vi "ReadDefaultConfigurationFile.vi"(8 "error in (no error)":errorcluster, 11 "SMO.UI.MAUI in":refnum<class "SMO.UI.MAUI.lvclass">) -> (0 "error out":errorcluster, 2 "Default Data":T1, 3 "SMO.UI.MAUI out":refnum<class "SMO.UI.MAUI.lvclass">)   [LabVIEW 2020, in "SMO.UI.MAUI.lvclass"]
doc: "Reads the framework's default configuration data. The configuration file is located at %PublicApplicationData%\\maui\\maui_framework\\resource\\default.ini."
uses:
  SMO.UI.MAUI.lvclass
  Typedefs/DefaultConfiguration.ctl
  <vilib>/Utility/config.llb/NI_LVConfig.lvlib
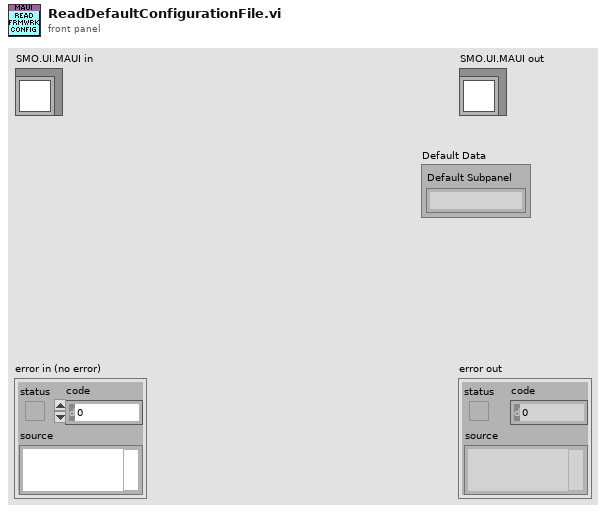
[diagram p1: front panel]
types:
  T1 = typedef "SMO.UI.MAUI.lvclass/DefaultConfiguration.ctl" = cluster{"Default Subpanel":string}
  T2 = typedef "NI_LVConfig.lvlib/Config Data RefNum.ctl" = refnum<k1>
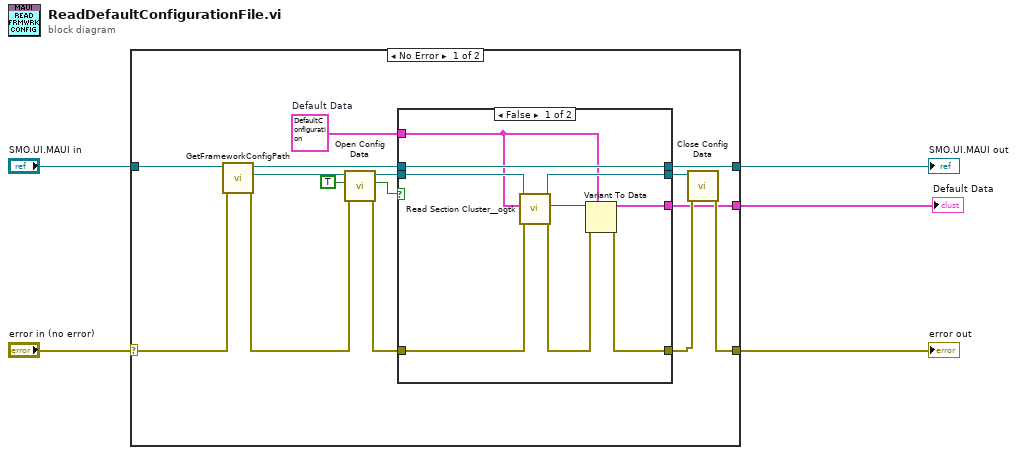
[diagram p0: block diagram]
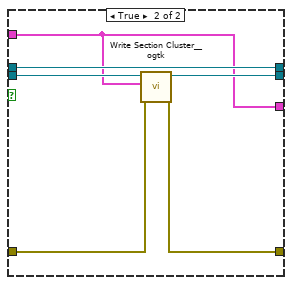
[diagram p2: hidden frame]
diagram:
  n1 = case shown="No Error" "error in (no error)" {
    selector: "error in (no error)" -> [w20 w37]
    tunnel: [w16 w37] -> w4
    tunnel: [w11 w36] -> w2
    tunnel: "SMO.UI.MAUI in" -> [w15 w36]
    tunnel: [w6 _] -> w1
    frame No Error {
      w8 = T1 {"Default Subpanel"="C:\\Program Files (x86)\\National Instruments\\LabVIEW 2020\\templates\\JKI\\JKI SMO\\LevyLab\\SMO.UI.Embedded.Basic.lvclass"}  # Default Data
      n2 = call "GetFrameworkConfigPath.vi"("error in (no error)"=w20, "SMO.UI.MAUI in"=w15) -> ("error out"=w19:errorcluster, "Path"=w13:path, "SMO.UI.MAUI out"=w12:refnum<class "SMO.UI.MAUI.lvclass">)  [unwired: 7 in]
      n3 = call <vilib>:"Open Config Data.vi"("error in (no error)"=w19, "create file if necessary (T)"=TRUE, "configuration file path"=w13) -> ("error out"=w18:errorcluster, "file created?"=w10:bool, "refnum"=w9:T2)  [unwired: 6 in]
      n4 = case shown="False" w10 {
        tunnel: w12 -> [w26 w33]
        tunnel: [w26 w33] -> w11
        tunnel: [w27 w35] -> w17
        tunnel: w18 -> [w29 w34]
        tunnel: w9 -> [w25 w32]
        tunnel: [w24 w31] -> w7
        tunnel: w8 -> [w22 w30]
        tunnel: [w21 w30] -> w6
        frame False {
          n5 = call <userlib>:"Read Section Cluster__ogtk.vi"("error in (no error)"=w29, "Section Formatted Cluster Type"=w22, "refnum"=w25) -> ("error out"=w28:errorcluster, "Section Formatted Cluster"=w23:variant, "dup refnum"=w24:T2)  [unwired: 4 in, 2 out]
          n6 = Variant To Data(error in=w28, type=w22, Variant=w23) -> (data=w21:T1, error out=w27:errorcluster)
        }
        frame True {
          n7 = call <userlib>:"Write Section Cluster__ogtk.vi"("error in (no error)"=w34, "Section Formatted Cluster"=w30, "refnum"=w32) -> ("error out"=w35:errorcluster, "dup refnum"=w31:T2)  [unwired: 7 in]
        }
      }
      n8 = call <vilib>:"Close Config Data.vi"("error in (no error)"=w17, "refnum"=w7) -> ("error out"=w16:errorcluster)  [unwired: 8 in, 1 out]
    }
    frame Error {
    }
  }
  "error out" <- w4
  "SMO.UI.MAUI out" <- w2
  "Default Data" <- w1
